vi "Chart Window LV2012.vi"(11 "Numeric":dbl) -> (3 "This VI":refnum<vi>)   [LabVIEW 2016]
panel:
  in  "Close This Window":bool
  out "Waveform Chart":dbl(graph)
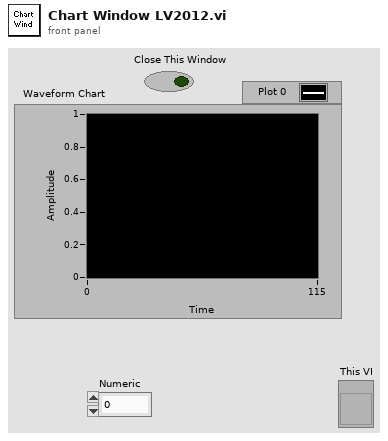
[diagram p1: front panel]
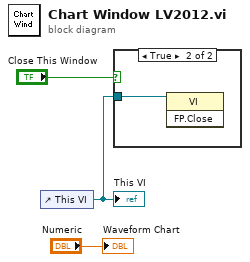
[diagram p0: block diagram]
diagram:
  n1 = control-ref of="This VI"() -> (w2:refnum<vi>)
  "This VI" <- w2
  n2 = case shown="True" "Close This Window" {
    tunnel: w2 -> [_ w4]
    frame False {
    }
    frame True {
      n3 = invoke class="VI" method="FP.Close"(reference=w4) -> ()  [unwired: 2 in, 3 out]
    }
  }
  "Waveform Chart" <- "Numeric"
